vi "Extended User Data.vi"(7 "Action (1: Write Data)":i32(ring)=1 items=["Read Data", "Write Data", "Clear Data", "Clear ALL Data"], 8 "error in (no error)":errorcluster, 10 "User Data In":T1 {"DPO MSO Series Model" items=["DPO4104", "DPO4054", "DPO4034", "DPO4032", "MSO4104", "MSO4054", "MSO4034", "MSO4032", "DPO3054", "DPO3052", "DPO3034", "DPO3032", "DPO3014", "DPO3012", "MSO3012", "MSO3014", "MSO3032", "MSO3034", "MSO3052", "MSO3054", "DPO2024", "DPO2014", "DPO2012", "DPO2002", "MSO2024", "MSO2014", "MSO2012", "MSO2002", "MDO4104-6", "MDO4104-3", "MDO4054-6", "MDO4054-3", "DPO4102", "MSO4102", "DPO2022B", "DPO2012B", "DPO2002B", "DPO2024B", "DPO2004B", "DPO2014B", "MSO2024B", "MSO2014B", "MSO2004B", "MSO2012B", "MSO2022B", "MSO2002B", "MDO4014B-3", "MDO4034B-3", "MDO4054B-3", "MDO4054B-6", "MDO4104B-3", "MDO4104B-6", "DPO4034B", "DPO4054B", "DPO4102B", "DPO4102B-L", "DPO4104B", "DPO4104B-L", "MSO4034B", "MSO4054B", "MSO4102B", "MSO4102B-L", "MSO4104B", "MSO4104B-L", "MDO3012", "MDO3022", "MDO3032", "MDO3052", "MDO3102", "MDO3014", "MDO3024", "MDO3034", "MDO3054", "MDO3104", "MDO4024C", "MDO4034C", "MDO4054C", "MDO4104C"]}, 11 "VISA resource name":refnum<visa-resource-name>) -> (0 "error out":errorcluster, 2 "User Data Out":T1 {"DPO MSO Series Model" items=["DPO4104", "DPO4054", "DPO4034", "DPO4032", "MSO4104", "MSO4054", "MSO4034", "MSO4032", "DPO3054", "DPO3052", "DPO3034", "DPO3032", "DPO3014", "DPO3012", "MSO3012", "MSO3014", "MSO3032", "MSO3034", "MSO3052", "MSO3054", "DPO2024", "DPO2014", "DPO2012", "DPO2002", "MSO2024", "MSO2014", "MSO2012", "MSO2002", "MDO4104-6", "MDO4104-3", "MDO4054-6", "MDO4054-3", "DPO4102", "MSO4102", "DPO2022B", "DPO2012B", "DPO2002B", "DPO2024B", "DPO2004B", "DPO2014B", "MSO2024B", "MSO2014B", "MSO2004B", "MSO2012B", "MSO2022B", "MSO2002B", "MDO4014B-3", "MDO4034B-3", "MDO4054B-3", "MDO4054B-6", "MDO4104B-3", "MDO4104B-6", "DPO4034B", "DPO4054B", "DPO4102B", "DPO4102B-L", "DPO4104B", "DPO4104B-L", "MSO4034B", "MSO4054B", "MSO4102B", "MSO4102B-L", "MSO4104B", "MSO4104B-L", "MDO3012", "MDO3022", "MDO3032", "MDO3052", "MDO3102", "MDO3014", "MDO3024", "MDO3034", "MDO3054", "MDO3104", "MDO4024C", "MDO4034C", "MDO4054C", "MDO4104C"]}, 3 "VISA resource name out":refnum<visa-resource-name>)   [LabVIEW 2016, in "Tektronix DPO MSO 2000 4000 Series.lvlib"]
doc: "You can use this VI to perform an action on current VI settings, such as write, read, clear and clear all."
uses:
  Tektronix DPO MSO 2000 4000 Series.lvlib
  Extended User Data.ctl
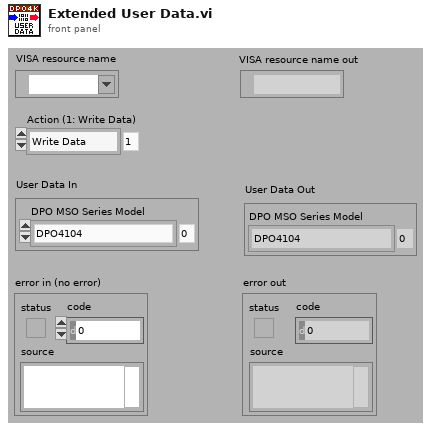
[diagram p1: front panel]
types:
  T1 = typedef "Tektronix DPO MSO 2000 4000 Series.lvlib/Extended User Data.ctl" = cluster{"DPO MSO Series Model":u16}
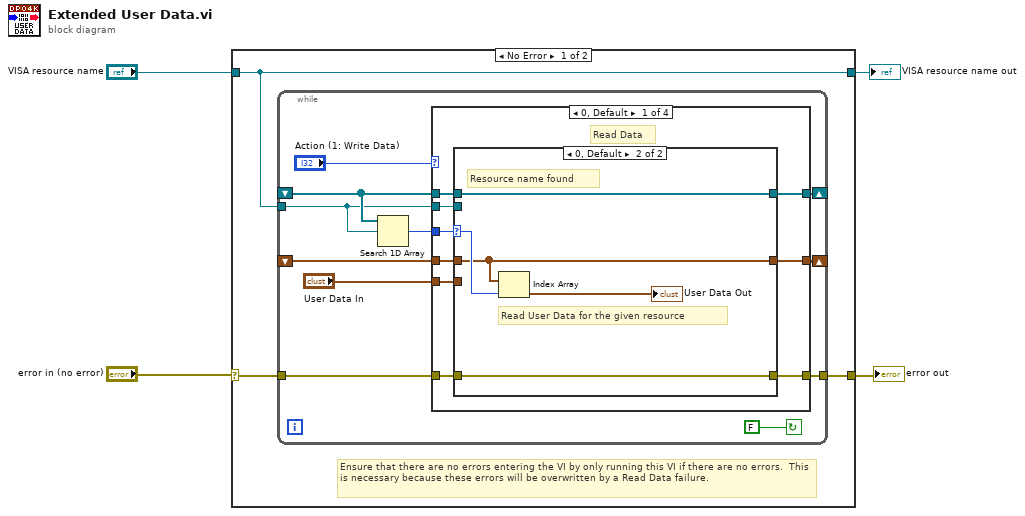
[diagram p0: block diagram]
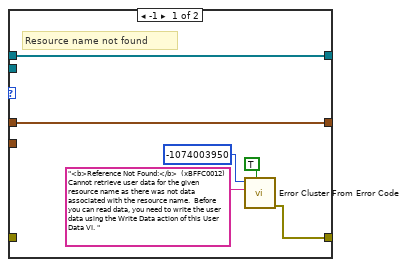
[diagram p2: hidden frame]
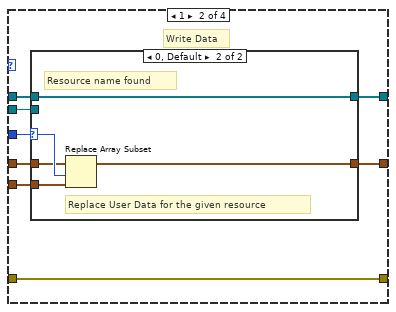
[diagram p3: hidden frame]
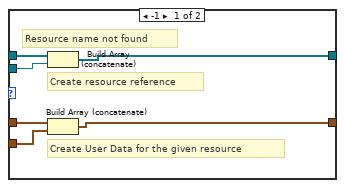
[diagram p4: hidden frame]
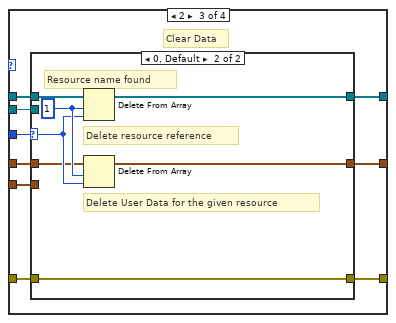
[diagram p5: hidden frame]
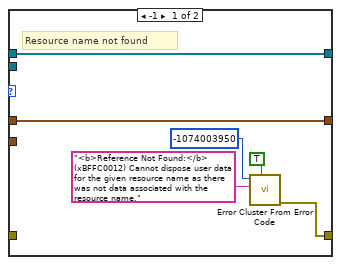
[diagram p6: hidden frame]
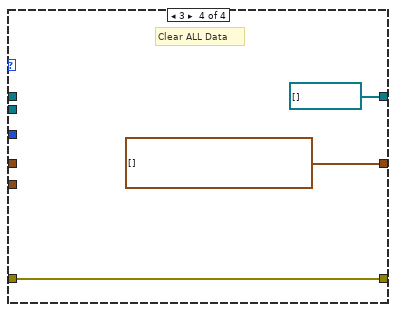
[diagram p7: hidden frame]
diagram:
  n1 = case shown="No Error" "error in (no error)" {
    selector: "error in (no error)" -> [w6 w84]
    tunnel: "VISA resource name" -> [w5 w83]
    tunnel: [w7 w84] -> w2
    tunnel: [w5 w83] -> w1
    frame No Error {
      # "Ensure that there are no errors entering the VI by only running this VI if there are no errors.  This is necessary because these errors will be overwritten by a Read Data failure."
      n2 = while {
        shift-right: [w16] -> _
        shift-left: _ -> [w17]
        tunnel: w5 -> [w15]
        tunnel: w6 -> [w13]
        tunnel: [w12] -> w7
        shift-right: [w9] -> _
        shift-left: _ -> [w8]
        stop <- FALSE continue-if-true
        n3 = Search 1D Array(1D array=w17, element=w15) -> (index of element=w18:i32)  [unwired: 1 out]
        n4 = case shown="0, Default" "Action (1: Write Data)" {
          tunnel: "User Data In" -> [w27 w46 w66 _]
          tunnel: w18 -> [w26 w45 w65 _]
          tunnel: w17 -> [w25 w44 w64 _]
          tunnel: [w24 w43 w63 refnum<visa-resource-name>[] []] -> w16
          tunnel: w15 -> [w23 w42 w62 _]
          tunnel: w13 -> [w21 w41 w60 w81]
          tunnel: [w22 w41 w61 w81] -> w12
          tunnel: [w20 w40 w58 T1[] []] -> w9
          tunnel: w8 -> [w19 w39 w59 _]
          frame 0, Default {
            # "Read Data"
            n5 = case shown="0, Default" w26 {
              selector: w26 -> [_ w38]
              tunnel: w27 -> [_ _]
              tunnel: w25 -> [w33 w37]
              tunnel: [w33 w37] -> w24
              tunnel: w23 -> [_ _]
              tunnel: [w32 w36] -> w22
              tunnel: w21 -> [_ w36]
              tunnel: [w28 w34] -> w20
              tunnel: w19 -> [w28 w34]
              frame -1 {
                # "Resource name not found"
                n6 = call <vilib>:"Error Cluster From Error Code.vi"("show call chain? (False)"=TRUE, "error message (\"\")"="<b>Reference Not Found:</b>  (xBFFC0012) Cannot retrieve user data for the given resource name as there was not data associated with the resource name.  Before you can read data, you need to write the user data using the Write Data action of this User Data VI. ", "error code (0)"=-1074003950 ("Code")) -> ("error out"=w32:errorcluster)  [unwired: 1 in, 5 out]
              }
              frame 0, Default {
                # "Read User Data for the given resource"
                # "Resource name found"
                n7 = Index Array(array=w34, index=w38) -> (element=→"User Data Out":T1)
              }
            }
          }
          frame 1 {
            # "Write Data"
            n8 = case shown="0, Default" w45 {
              selector: w45 -> [_ w57]
              tunnel: w46 -> [w51 w53]
              tunnel: w44 -> [w52 w56]
              tunnel: [w49 w56] -> w43
              tunnel: w42 -> [w50 _]
              tunnel: [w48 w55] -> w40
              tunnel: w39 -> [w47 w54]
              frame -1 {
                # "Create resource reference"
                # "Create User Data for the given resource"
                # "Resource name not found"
                n9 = Build Array (concatenate)(w52, w50) -> (w49:refnum<visa-resource-name>[])
                n10 = Build Array (concatenate)(w47, w51) -> (w48:T1[])
              }
              frame 0, Default {
                # "Replace User Data for the given resource"
                # "Resource name found"
                n11 = Replace Array Subset(array=w54, new element=w53, index=w57) -> (w55:T1[])
              }
            }
          }
          frame 2 {
            # "Clear Data"
            n12 = case shown="0, Default" w65 {
              selector: w65 -> [_ w74]
              tunnel: w66 -> [_ _]
              tunnel: [w67 w79] -> w58
              tunnel: w64 -> [w72 w77]
              tunnel: [w72 w76] -> w63
              tunnel: w62 -> [_ _]
              tunnel: [w71 w78] -> w61
              tunnel: w60 -> [_ w78]
              tunnel: w59 -> [w67 w73]
              frame -1 {
                # "Resource name not found"
                n13 = call <vilib>:"Error Cluster From Error Code.vi"("show call chain? (False)"=TRUE, "error message (\"\")"="<b>Reference Not Found:</b>  (xBFFC0012) Cannot dispose user data for the given resource name as there was not data associated with the resource name.", "error code (0)"=-1074003950 ("Code")) -> ("error out"=w71:errorcluster)  [unwired: 1 in, 5 out]
              }
              frame 0, Default {
                w75 = 1 ("length")
                # "Delete resource reference"
                # "Delete User Data for the given resource"
                # "Resource name found"
                n14 = Delete From Array(array=w77, length=w75, index=w74) -> (array with subset deleted=w76:refnum<visa-resource-name>[])  [unwired: 1 out]
                n15 = Delete From Array(array=w73, length=w75, index=w74) -> (array with subset deleted=w79:T1[])  [unwired: 1 out]
              }
            }
          }
          frame 3 {
            # "Clear ALL Data"
          }
        }
      }
    }
    frame Error {
    }
  }
  "VISA resource name out" <- w1
  "error out" <- w2
